vi "CSM - Request CSM to Post Message.vi"(4 "Immediately? (F)":bool, 6 "Without Reply? (F)":bool, 7 "Module Name":string, 8 "Error In (No Error)":errorcluster, 9 "Target Module (\"\" By Default)":string, 10 "Arguments (\"\")":string, 11 "State":string) -> (0 "error out":errorcluster)   [LabVIEW 2017, in "Communicable State Machine.lvlib"]
doc: "### CSM - Request CSM to Post Message.vi\n\nRequest CSM to send a message. Typically used for functional loops running in parallel with CSM, these loops complete the full module functionality together with CSM.\n\n-- <b>Controls</b> --\n- <b>Module Name</b>: CSM sending the status\n- <b>Status</b>: Status to be broadcasted\n- <b>Arguments (\"\")</b>: Parameters of the status to be broadcasted\n- <b>Target Module</b>: Target module"
uses:
  Communicable State Machine.lvlib
  _Support/CSMQ/_CSMOFGVOPER.ctl
  _Support/Typedef/_Cross CSM State Data.ctl
  _Support/Typedef/_CSM_MSG_TYPE.ctl
  _Support/Typedef/_Cross CSM State Response.ctl
  _Support/Typedef/_CSM_Response Source Message.ctl
  _Shared/CSM Shared.lvlib
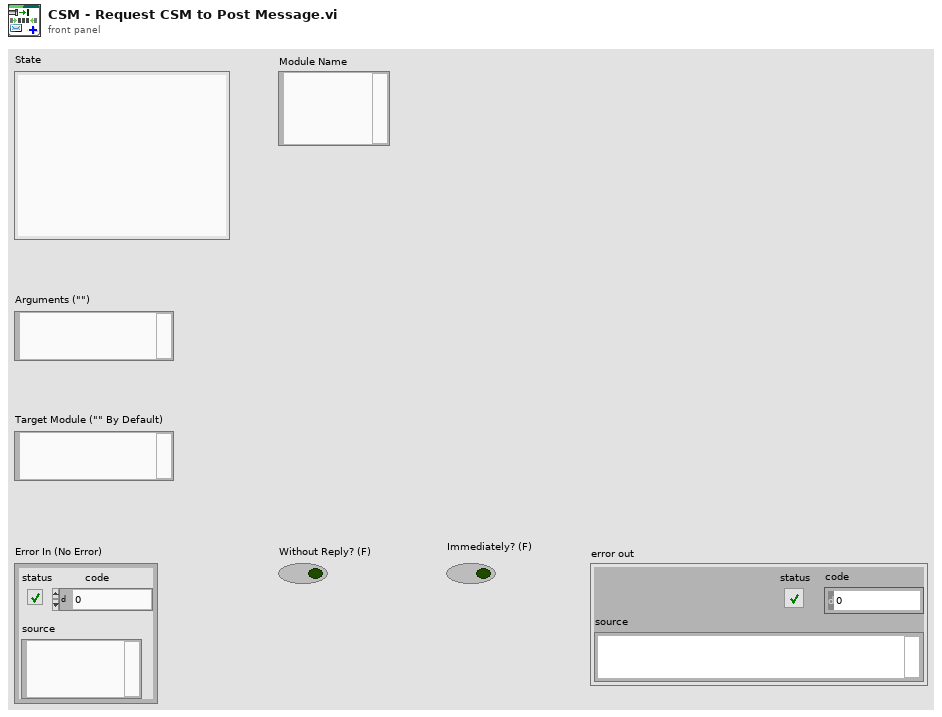
[diagram p1: front panel]
types:
  T1 = typedef "Communicable State Machine.lvlib/_CSM_MSG_TYPE.ctl" = enum16{"Sync Message(-@)", "Async Message(->)", "Async without Response(->|)", "Async Response", "Broadcast(-><all>)", "Broadcast(-><status>)", "Broadcast(-><interrupt>)", "Append to JKISM States", "Append to JKISM States(High Priority)", "Broadcast(-><state>)"}
  T2 = typedef "Communicable State Machine.lvlib/_Cross CSM State Data.ctl" = cluster{"Msg Type":T1, "state":string, "args":string, "source":string, "RespQ":refnum<queue>, "Response For Message":T3, "Target":string}
  T3 = typedef "Communicable State Machine.lvlib/_CSM_Response Source Message.ctl" = cluster{"‘State":string, "’Arguments":string, "’Error":errorcluster}
  T4 = typedef "Communicable State Machine.lvlib/_CSMOFGVOPER.ctl" = enum16{"Create If not Exist", "Get By Name", "List", "Check If Name Exists", "Release", "Module Status", "Create Status Event Handler", "Destroy Status Event Handler", "Clear Invalid Objs"}
  T5 = typedef "Communicable State Machine.lvlib/_CSMObj.ctl" = cluster{"info":T6, "Refs":T8}
  T6 = typedef "Communicable State Machine.lvlib/_CSMObj-Info.ctl" = cluster{"Module Name":string, "Requested Name":string, "Group Name":string, "Mode":T7, "Allowed Messages":string[]}
  T7 = typedef "Communicable State Machine.lvlib/_CSM_MODE.ctl" = enum16{"Not Exist", "Stand Alone", "CSM", "Worker", "Worker Agent", "Chain Node", "Chain"}
  T8 = typedef "Communicable State Machine.lvlib/_CSMObj-Refs.ctl" = cluster{"WatchDogQ":refnum<queue>, "CSMDataDVR":refnum<data-value>, "Queue":T9, "GroupDataDVR":refnum<data-value>, "TagMap":refnum<data-value>, "ExitEvent":refnum<user-event>, "NewStateEvent":refnum<user-event>, "StatusChangeEvent":refnum<user-event>}
  T9 = typedef "Communicable State Machine.lvlib/Priority Queue.ctl" = cluster{"HPriorityQ":refnum<queue>, "LowPriorityQ":refnum<queue>}
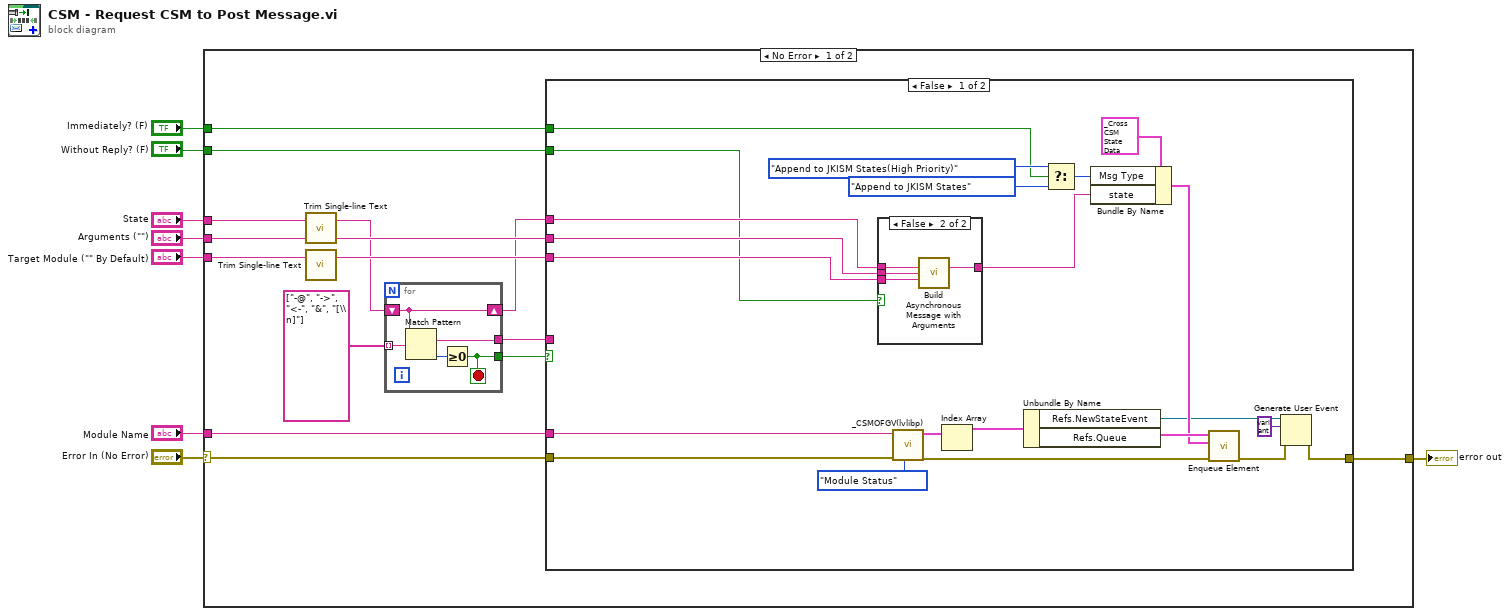
[diagram p0: block diagram]
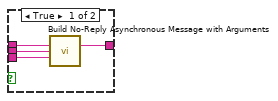
[diagram p2: hidden frame]
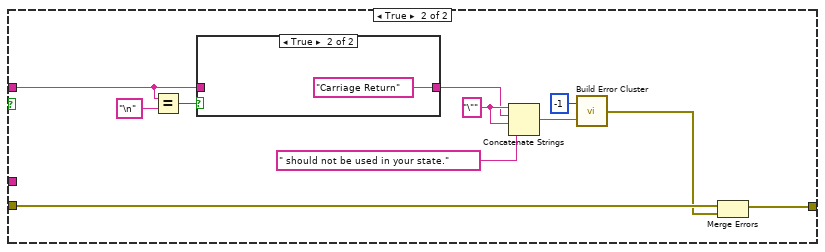
[diagram p3: hidden frame]
diagram:
  n1 = case shown="No Error" "Error In (No Error)" {
    selector: "Error In (No Error)" -> [w20 w71]
    tunnel: "State" -> [w17 _]
    tunnel: [w21 w71] -> w6
    tunnel: "Arguments (\"\")" -> [w18 _]
    tunnel: "Target Module (\"\" By Default)" -> [w22 _]
    tunnel: "Module Name" -> [w16 _]
    tunnel: "Without Reply? (F)" -> [w15 _]
    tunnel: "Immediately? (F)" -> [w9 _]
    frame No Error {
      n2 = call "Trim Single-line Text.vi"("single-line text"=w17) -> ("trimed text"=w10:string)  [unwired: 2 in]
      n3 = call "Trim Single-line Text.vi"("single-line text"=w22) -> ("trimed text"=w19:string)  [unwired: 2 in]
      n4 = for {
        shift-right: [w70] -> w13
        shift-left: w10 -> [w70]
        tunnel: string[] ["-@", "->", "<-", "&", "[\\n]"] -> [w69] mode=indexing
        tunnel: [w67] -> w11
        tunnel: [w66] -> w12
        stop <- w66 stop-if-true
        n5 = Match Pattern(string=w70, regular expression=w69) -> (match substring=w67:string, offset past match=w68:i32)  [unwired: 1 in, 2 out]
        n6 = Greater Or Equal To 0?(x=w68) -> (x >= 0?=w66:bool)
      }
      n7 = case shown="False" w12 {
        tunnel: w18 -> [w29 _]
        tunnel: w19 -> [w28 _]
        tunnel: [w33 w55] -> w21
        tunnel: w20 -> [w37 w56]
        tunnel: w13 -> [w30 _]
        tunnel: w11 -> [_ w53]
        tunnel: w16 -> [w35 _]
        tunnel: w15 -> [w23 _]
        tunnel: w9 -> [w24 _]
        frame False {
          n8 = case shown="False" w23 {
            tunnel: w30 -> [w48 w52]
            tunnel: w29 -> [w47 w51]
            tunnel: w28 -> [w46 w50]
            tunnel: [w45 w49] -> w27
            frame True {
              n9 = call "Build No-Reply Asynchronous Message with Arguments.vi"("State With Arguments"=w48, "Arguments (\"\")"=w47, "Target Module (\"\")"=w46) -> ("CSM Message String"=w45:string)  [unwired: 12 in]
            }
            frame False {
              n10 = call "Build Asynchronous Message with Arguments.vi"("State With Arguments"=w52, "Arguments (\"\")"=w51, "Target Module (\"\")"=w50) -> ("CSM Message String"=w49:string)  [unwired: 12 in]
            }
          }
          n11 = call "_CSMOFGV(lvlibp).vi"("Operation"=_CSMOFGVOPER."Module Status", "Error In"=w37, "Name (\"\" to Use UUID) In"=w35) -> ("error out"=w38:errorcluster, "Array"=w43:T5[])  [unwired: 6 in, 1 out]
          n12 = Index Array(array=w43) -> (element=w42:T5)  [unwired: 1 in]
          n13 = Unbundle By Name(w42) -> ("Refs.NewStateEvent"=w32:refnum<user-event>, "Refs.Queue"=w41:T9)
          n14 = Select(t=_CSM_MSG_TYPE."Append to JKISM States(High Priority)" ("Msg Type"), s=w24, f=_CSM_MSG_TYPE."Append to JKISM States" ("Msg Type")) -> (s? t:f=w34:T1)
          n15 = Bundle By Name(cluster=T2 {"Msg Type"=enum."Sync Message(-@)", "state"="", "args"="", "source"="", "RespQ"=refnum, "Response For Message"={"‘State"="", "’Arguments"="", "’Error"={"status"=FALSE, "code"=0, "source"=""}}, "Target"=""} ("element"), "Msg Type"=w34, "state"=w27) -> (w39:T2)
          n16 = call "Enqueue Element.vi"("error in (no error)"=w38, "Cross JKI State Machine State"=w39, "Priority Queue"=w41) -> ("error out"=w36:errorcluster)  [unwired: 7 in, 1 out]
          n17 = Generate User Event(user event=w32, event data cluster=variant ("event data"), error in=w36) -> (error out=w33:errorcluster)  [unwired: 1 in, 1 out]
        }
        frame True {
          w60 = "\"" ("string")
          n18 = Equal?(x=w53, y="\n" ("regular expression")) -> (x = y?=w57:bool)
          n19 = case shown="True" w57 {
            tunnel: [w64 "Carriage Return" ("State")] -> w59
            tunnel: w53 -> [w64 _]
            frame False {
            }
            frame True {
            }
          }
          n20 = Concatenate Strings(w60, w59, w60, " should not be used in your state." ("String to Prepend to source (\"\")")) -> (w61:string)
          n21 = call "Build Error Cluster.vi"("String to Prepend to Source (\"\")"=w61, "Code"=-1 ("code")) -> ("error out"=w54:errorcluster)
          n22 = Merge Errors(w56, w54) -> (w55:errorcluster)
        }
      }
    }
    frame Error {
    }
  }
  "error out" <- w6
